vi "Read Crypto Library Path.vi"(8 "error in (no error)":errorcluster, 11 "SSL-Lib in":refnum<class "SSL-Lib.lvclass">) -> (0 "error out":errorcluster, 2 "Crypto Library Path":path=path "C:/Program Files (x86)/National Instruments/Shared/nissl/NIlibeay32.dll", 3 "SSL-Lib out":refnum<class "SSL-Lib.lvclass">)   [LabVIEW 2013, in "SSL_Lib.lvlib" / "SSL-Lib.lvclass"]
uses:
  SSL-Lib.lvclass
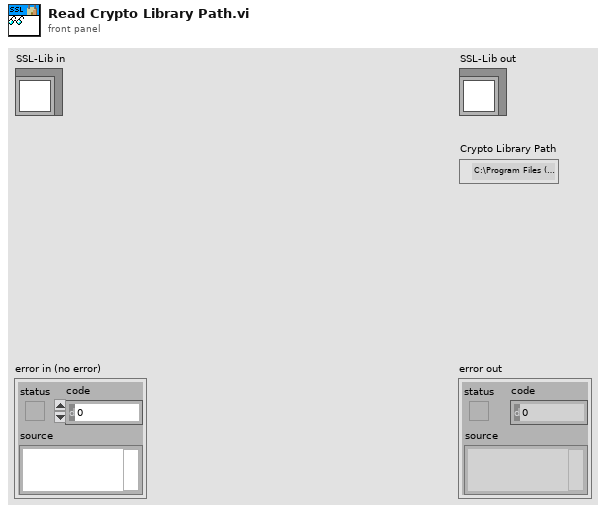
[diagram p1: front panel]
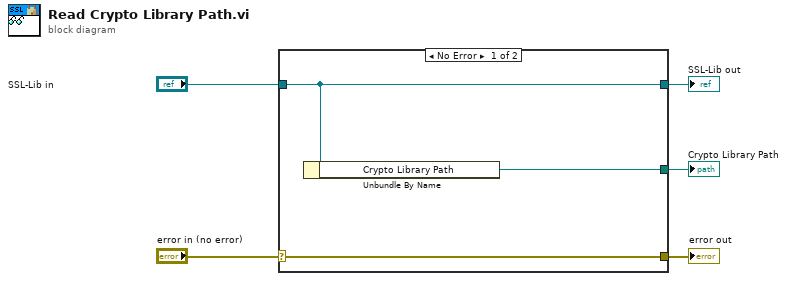
[diagram p0: block diagram]
diagram:
  n1 = case shown="No Error" "error in (no error)" {
    selector: "error in (no error)" -> [w8 w9]
    tunnel: [w8 w9] -> w4
    tunnel: [w7 w10] -> w2
    tunnel: "SSL-Lib in" -> [w7 w10]
    tunnel: [w6 _] -> w1
    frame No Error {
      n2 = Unbundle By Name(w7) -> ("Crypto Library Path"=w6:path)
    }
    frame Error {
    }
  }
  "error out" <- w4
  "SSL-Lib out" <- w2
  "Crypto Library Path" <- w1
